vi "ResultLoadPrompt.vi"(0 "Path":path) -> (1 "selected path":path, 2 "cancel?":bool)   [LabVIEW 2020]
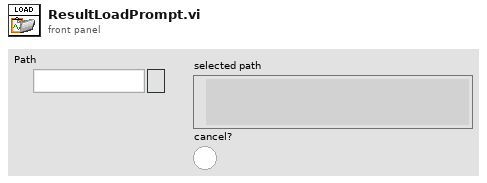
[diagram p1: front panel]
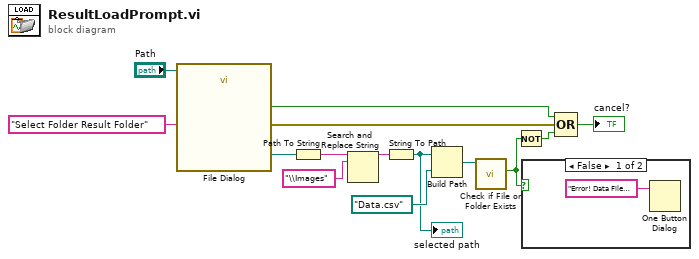
[diagram p0: block diagram]
diagram:
  n1 = call "File Dialog"("start path"="Path", "prompt"="Select Folder Result Folder") -> ("selected path"=w6:path, "cancelled"=w13:bool, "error out"=w14:errorcluster)  [unwired: 10 in, 1 out]
  n2 = Path To String(path=w6) -> (string=w9:string)
  n3 = Search and Replace String(input string=w9, search string="\\Images") -> (result string=w7:string)  [unwired: 6 in, 3 out]
  n4 = String To Path(string=w7) -> (path=w1:path)
  "selected path" <- w1
  n5 = Build Path(base path=w1, name or relative path=path "Data.csv") -> (appended path=w4:path)
  n6 = call <vilib>:"Check if File or Folder Exists.vi"("path"=w4) -> ("file or folder exists?"=w2:bool)  [unwired: 8 in, 2 out]
  n7 = Not(x=w2) -> (.not. x?=w3:bool)
  n8 = case shown="False" w2 {
    frame False {
      n9 = One Button Dialog(message="Error! Data File not found in selected folder") -> ()  [unwired: 1 in, 1 out]
    }
    frame True {
    }
  }
  n10 = Compound Arithmetic op=OR(w13, w14, w3) -> (→"cancel?":bool)
